vi "Dequeue Performance Test.vi"() -> ()   [LabVIEW 2021]
panel:
  out "x-y":dbl format="%#_6p"
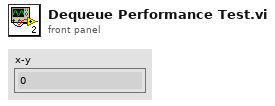
[diagram p1: front panel]
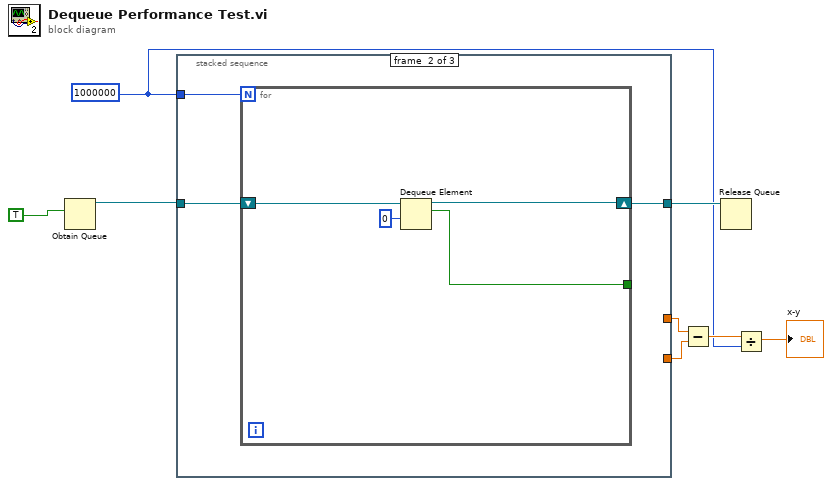
[diagram p0: block diagram]
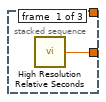
[diagram p2: hidden frame]
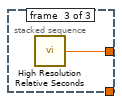
[diagram p3: hidden frame]
diagram:
  w1 = 1000000
  n1 = Obtain Queue(element data type=TRUE) -> (queue out=w8:refnum<queue>)  [unwired: 4 in, 2 out]
  n2 = stacked-sequence {
    tunnel: w8 -> [_ w12 _]
    tunnel: [_ w11 _] -> w6
    tunnel: [w9 _ _] -> w5
    tunnel: [_ _ w17] -> w4
    tunnel: w1 -> [_ w10 _]
    frame #0 {
      n3 = call <vilib>:"High Resolution Relative Seconds.vi"() -> ("relative seconds"=w9:dbl)
    }
    frame #1 {
      n4 = for {
        N: w10 -> [_]
        shift-right: [w15] -> w11
        shift-left: w12 -> [w16]
        tunnel: [w14] -> _
        n5 = Dequeue Element(queue=w16, timeout in ms (-1)=0) -> (queue out=w15:refnum<queue>, element=w14:bool)  [unwired: 1 in, 2 out]
      }
    }
    frame #2 {
      n6 = call <vilib>:"High Resolution Relative Seconds.vi"() -> ("relative seconds"=w17:dbl)
    }
  }
  n7 = Subtract(x=w4, y=w5) -> (x-y=w3:dbl)
  n8 = Release Queue(queue=w6) -> ()  [unwired: 2 in, 3 out]
  n9 = Divide(x=w3, y=w1) -> (x/y=→"x-y":dbl)
